vi "Measure.vi"(8 "error in":errorcluster, 11 "PowerSupply in":refnum<class "PowerSupply.lvclass">) -> (0 "error out":errorcluster, 3 "PowerSupply out":refnum<class "PowerSupply.lvclass">)   [LabVIEW 2019, in "PowerSupply.lvlib" / "PowerSupply.lvclass"]
uses:
  Library/PowerSupply.lvclass
  builds/Instruments/Instruments.lvlibp/Library/Instruments.lvclass
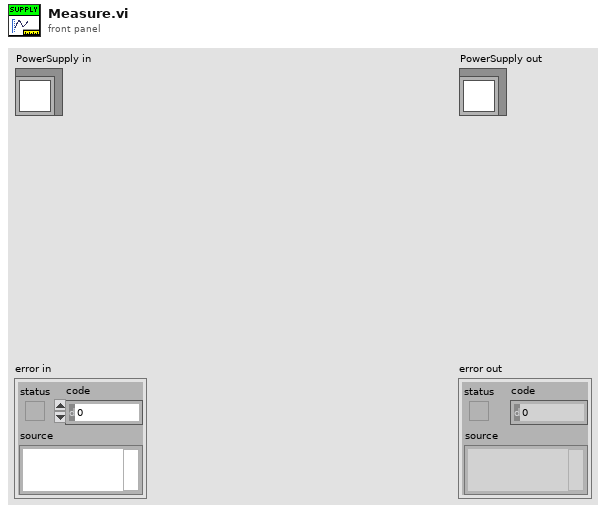
[diagram p1: front panel]
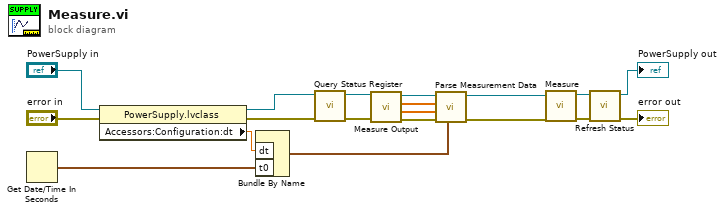
[diagram p0: block diagram]
diagram:
  n1 = Get Date/Time In Seconds() -> (seconds since 1Jan1904=w12:timestamp)
  n2 = property class="PowerSupply.lvclass"(reference="PowerSupply in", error in="error in") -> (reference out=w8:refnum<class "PowerSupply.lvclass">, error out=w9:errorcluster, "Accessors:Configuration:dt"=w13:dbl)
  n3 = Bundle By Name("dt"=w13, "t0"=w12) -> (w3:waveform(dbl))  [unwired: 1 in]
  n4 = call-dynamic "Query Status Register.vi"("error in (no error)"=w9, "PowerSupply in"=w8) -> ("error out"=w11:errorcluster, "PowerSupply out"=w10:refnum<class "PowerSupply.lvclass">)  [unwired: 8 in]
  n5 = call-dynamic "Measure Output.vi"("error in (no error)"=w11, "PowerSupply in"=w10) -> ("error out"=w6:errorcluster, "Current"=w2:dbl[], "Voltage"=w1:dbl[], "PowerSupply out"=w7:refnum<class "PowerSupply.lvclass">)  [unwired: 6 in]
  n6 = call "Parse Measurement Data.vi"("Waveform Template"=w3, "error in"=w6, "Current"=w2, "Voltage"=w1, "PowerSupply in"=w7) -> ("error out"=w4:errorcluster, "PowerSupply out"=w5:refnum<class "PowerSupply.lvclass">)  [unwired: 5 in]
  n7 = call-parent "Measure.vi"("error in"=w4, "Instruments in"=w5) -> ("error out"=w18:errorcluster, "Instruments out"=w19:refnum<class "PowerSupply.lvclass">)  [unwired: 8 in]
  n8 = call "Refresh Status.vi"("error in"=w18, "PowerSupply in"=w19) -> ("error out"=→"error out":errorcluster, "PowerSupply out"=→"PowerSupply out":refnum<class "PowerSupply.lvclass">)  [unwired: 8 in]
